vi "GetPersistentConfiguration.vi"(8 "ErrorIn":errorcluster, 9 "DataIn":variant, 11 "ReferenceIn":refnum<class "TraceWindow.lvclass">) -> (0 "ErrorOut":errorcluster, 1 "DataOut":variant, 3 "ReferenceOut":refnum<class "TraceWindow.lvclass">)   [LabVIEW 2021, in "TraceWindow.lvlib" / "TraceWindow.lvclass"]
uses:
  TraceWindow.lvclass
  Library_TAF_ApplicationFramework/TAFBaseGUI/TAFBaseGUI.lvclass
  TraceWindow.lvclass/TraceWindow.ctl
  C:/Localdata/Projects/TriekselSoft/TriekselsoftApplicationFramework/Source/.Externals/Library_TAF_ApplicationFramework/TAFBaseGUI/TAFBaseGUI.lvclass
  C:/Localdata/Projects/TriekselSoft/TriekselsoftApplicationFramework/Source/.Externals/Interface_UserInterface_IFrontPanel/IFrontPanel/IFrontPanel.lvclass
  C:/Localdata/Projects/TriekselSoft/TriekselsoftApplicationFramework/Source/IInterface/IInterface.lvclass
  C:/Localdata/Projects/TriekselSoft/TriekselsoftApplicationFramework/Source/.Externals/Interface_TAF_ITAFGUIActions/ITAFGUIActions/ITAFGUIActions.lvclass
  C:/Localdata/Projects/TriekselSoft/TriekselsoftApplicationFramework/Source/.Externals/Interface_Object_ICreateDestroy/ICreateDestroy/ICreateDestroy.lvclass
  C:/Localdata/Projects/TriekselSoft/TriekselsoftApplicationFramework/Source/.Externals/Interface_Object_IPersistentData/IPersistentData/IPersistentData.lvclass
  C:/Localdata/Projects/TriekselSoft/TriekselsoftApplicationFramework/Source/.Externals/Interface_TAF_ITAFObject/ITAFObject/ITAFObject.lvclass
  C:/Localdata/Projects/TriekselSoft/TriekselsoftApplicationFramework/Source/.Externals/Library_TAF_TraceWindow/TraceWindow/TraceWindow.lvclass
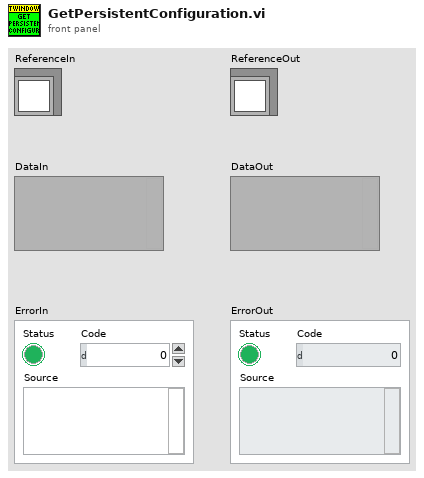
[diagram p1: front panel]
types:
  T1 = typedef "TraceWindow.lvlib/TraceWindow.lvclass/ObjectAttributes.ctl" = cluster{"Interfaces":cluster{"Dummys":refnum<class>}, "Locals":cluster{"MainGUIActive":refnum<queue>, "TraceQueue":refnum<queue>}, "Persistent":cluster{"OpenAtClosure":bool, "BufferSize":i32, "Startup":cluster{"OpenAtStartUp":bool, "OpenMinimized":bool}}}
  T2 = cluster{"OpenAtClosure":bool, "BufferSize":i32, "Startup":cluster{"OpenAtStartUp":bool, "OpenMinimized":bool}}
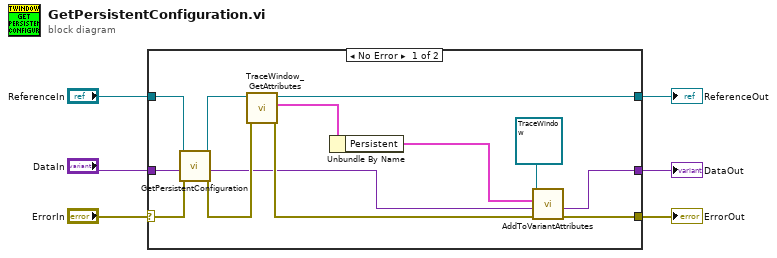
[diagram p0: block diagram]
diagram:
  n1 = case shown="No Error" "ErrorIn" {
    selector: "ErrorIn" -> [w19 w22]
    tunnel: [w17 w22] -> w5
    tunnel: [w14 w21] -> w3
    tunnel: "ReferenceIn" -> [w10 w21]
    tunnel: [w13 w20] -> w2
    tunnel: "DataIn" -> [w8 w20]
    frame No Error {
      n2 = call-parent "GetPersistentConfiguration.vi"("ErrorIn"=w19, "DataIn"=w8, "ReferenceIn"=w10) -> ("ErrorOut"=w16:errorcluster, "DataOut"=w7:variant, "ReferenceOut"=w9:refnum<class "TraceWindow.lvclass">)  [unwired: 6 in]
      n3 = call "TraceWindow_GetAttributes.vi"("ErrorIn"=w16, "ReferenceIn"=w9) -> ("ErrorOut"=w18:errorcluster, "Data"=w15:T1, "ReferenceOut"=w14:refnum<class "TraceWindow.lvclass">)  [unwired: 6 in, 1 out]
      n4 = Unbundle By Name(w15) -> ("Persistent"=w12:T2)
      n5 = call "AddToVariantAttributes.vi"("ErrorIn"=w18, "DataInIn"=w7, "PersistentData"=w12, "Object"=refnum<class "TraceWindow.lvclass"> refnum ("VerticalButtonBar")) -> ("ErrorOut"=w17:errorcluster, "DataInOut"=w13:variant)  [unwired: 6 in]
    }
    frame Error {
    }
  }
  "ErrorOut" <- w5
  "ReferenceOut" <- w3
  "DataOut" <- w2
